vi "ProbePlanShiftBias.vi"() -> ()   [LabVIEW 2013]
panel:
  in  "Strip Index":i32
  in  "X":dbl
  out "X_Bias":dbl
  in  "Region":i32
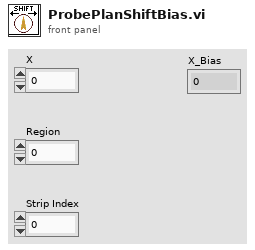
[diagram p1: front panel]
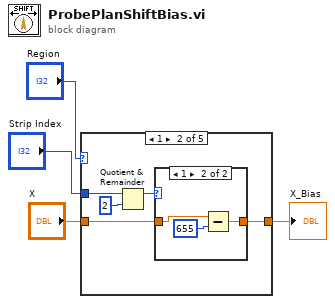
[diagram p0: block diagram]
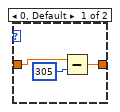
[diagram p3: hidden frame]
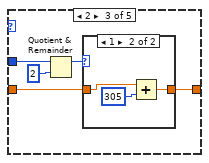
[diagram p4: hidden frame]
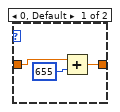
[diagram p5: hidden frame]
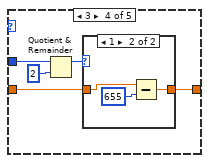
[diagram p6: hidden frame]
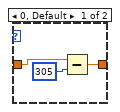
[diagram p7: hidden frame]
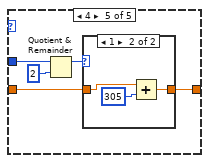
[diagram p8: hidden frame]
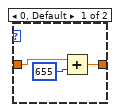
[diagram p9: hidden frame]
diagram:
  n1 = case shown="1" "Region" {
    tunnel: "X" -> [w5 w8 w18 w30 w40]
    tunnel: [w5 w6 w17 w28 w41] -> w2
    tunnel: "Strip Index" -> [_ w7 w20 w31 w39]
    frame 0, Default {
    }
    frame 1 {
      n2 = Quotient & Remainder(x=w7, y=2) -> (x-y*floor(x/y)=w9:i32)  [unwired: 1 out]
      n3 = case shown="1" w9 {
        tunnel: w8 -> [w13 w15]
        tunnel: [w11 w14] -> w6
        frame 0, Default {
          n4 = Subtract(x=w13, y=305) -> (x-y=w11:dbl)
        }
        frame 1 {
          n5 = Subtract(x=w15, y=655) -> (x-y=w14:dbl)
        }
      }
    }
    frame 2 {
      n6 = Quotient & Remainder(x=w20, y=2) -> (x-y*floor(x/y)=w19:i32)  [unwired: 1 out]
      n7 = case shown="1" w19 {
        tunnel: w18 -> [w23 w27]
        tunnel: [w22 w25] -> w17
        frame 0, Default {
          n8 = Add(x=w23, y=655) -> (x+y=w22:dbl)
        }
        frame 1 {
          n9 = Add(x=w27, y=305) -> (x+y=w25:dbl)
        }
      }
    }
    frame 3 {
      n10 = Quotient & Remainder(x=w31, y=2) -> (x-y*floor(x/y)=w29:i32)  [unwired: 1 out]
      n11 = case shown="1" w29 {
        tunnel: w30 -> [w35 w37]
        tunnel: [w33 w36] -> w28
        frame 0, Default {
          n12 = Subtract(x=w35, y=305) -> (x-y=w33:dbl)
        }
        frame 1 {
          n13 = Subtract(x=w37, y=655) -> (x-y=w36:dbl)
        }
      }
    }
    frame 4 {
      n14 = Quotient & Remainder(x=w39, y=2) -> (x-y*floor(x/y)=w42:i32)  [unwired: 1 out]
      n15 = case shown="1" w42 {
        tunnel: w40 -> [w45 w49]
        tunnel: [w44 w47] -> w41
        frame 0, Default {
          n16 = Add(x=w45, y=655) -> (x+y=w44:dbl)
        }
        frame 1 {
          n17 = Add(x=w49, y=305) -> (x+y=w47:dbl)
        }
      }
    }
  }
  "X_Bias" <- w2
